vi "UploadExperiments.vi"(8 "error in (no error)":errorcluster, 11 "DB in":refnum<class "DB.lvclass">) -> (0 "error out":errorcluster, 3 "DB out":refnum<class "DB.lvclass">)   [LabVIEW 2015, in "DB.lvclass"]
uses:
  DB.lvclass
  DB.lvclass/DB.ctl
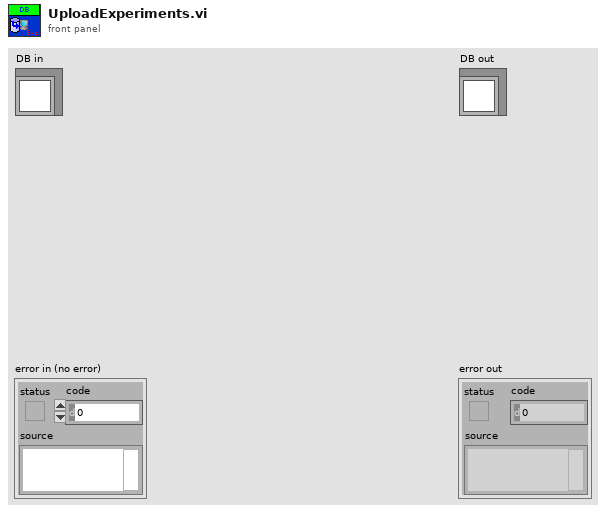
[diagram p1: front panel]
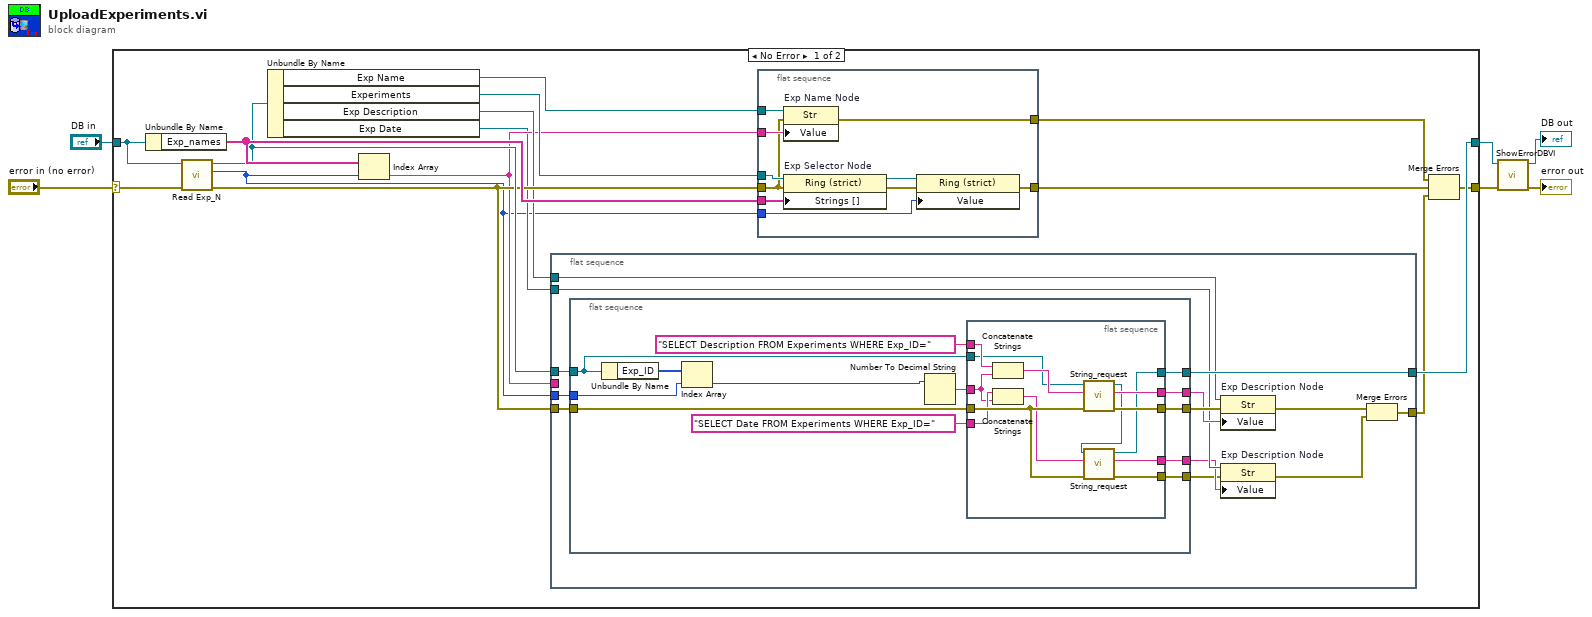
[diagram p0: block diagram]
diagram:
  n1 = case shown="No Error" "error in (no error)" {
    selector: "error in (no error)" -> [w21 w73]
    tunnel: [w14 w73] -> w6
    tunnel: [w15 w72] -> w5
    tunnel: "DB in" -> [w22 w72]
    frame No Error {
      n2 = Unbundle By Name(w22) -> ("Exp_names"=w19:string[])
      n3 = call "Read Exp_N.vi"("error in (no error)"=w21, "DB in"=w22) -> ("error out"=w13:errorcluster, "Exp_N"=w7:i16, "DB out"=w16:refnum<class "DB.lvclass">)  [unwired: 7 in]
      n4 = Unbundle By Name(w16) -> ("Exp Name"=w20:refnum<vi>, "Experiments"=w18:refnum<vi>, "Exp Description"=w12:refnum<vi>, "Exp Date"=w8:refnum<vi>)
      n5 = Index Array(array=w19, index=w7) -> (element=w9:string)
      n6 = flat-sequence {
        tunnel: w16 -> [w35]
        tunnel: [w45] -> w15
        tunnel: w13 -> [w37]
        tunnel: w12 -> [w43]
        tunnel: [w39] -> w10
        tunnel: w9 -> [_]
        tunnel: w8 -> [w41]
        tunnel: w7 -> [w34]
        frame #0 {
          n7 = flat-sequence {
            tunnel: [w58] -> w45
            tunnel: [w56] -> w44
            tunnel: [w55] -> w42
            tunnel: w37 -> [w54]
            tunnel: [w52] -> w36
            tunnel: w35 -> [w51]
            tunnel: w34 -> [w49]
            tunnel: [w46] -> w33
            frame #0 {
              n8 = Unbundle By Name(w51) -> ("Exp_ID"=w50:i16[])
              n9 = Index Array(array=w50, index=w49) -> (element=w48:i16)
              n10 = Number To Decimal String(number=w48) -> (decimal integer string=w47:string)  [unwired: 1 in]
              n11 = flat-sequence {
                tunnel: [w59] -> w58
                tunnel: "SELECT Description FROM Experiments WHERE Exp_ID=" ("SQL request") -> [w71]
                tunnel: [w69] -> w56
                tunnel: [w68] -> w55
                tunnel: w54 -> [w67]
                tunnel: "SELECT Date FROM Experiments WHERE Exp_ID=" ("SQL request") -> [w66]
                tunnel: [w64] -> w52
                tunnel: w51 -> [w63]
                tunnel: w47 -> [w62]
                tunnel: [w61] -> w46
                frame #0 {
                  n12 = Concatenate Strings(w71, w62) -> (w70:string)
                  n13 = Concatenate Strings(w66, w62) -> (w65:string)
                  n14 = call-dynamic "String_request.vi"("error in (no error)"=w67, "SQL request"=w70, "DB in"=w63) -> ("error out"=w69:errorcluster, "Result"=w68:string, "DB out"=w60:refnum<class "DB.lvclass">)  [unwired: 6 in]
                  n15 = call-dynamic "String_request.vi"("error in (no error)"=w67, "SQL request"=w65, "DB in"=w60) -> ("error out"=w61:errorcluster, "Result"=w64:string, "DB out"=w59:refnum<class "DB.lvclass">)  [unwired: 6 in]
                }
              }
            }
          }
          n16 = property on="Exp Description Node" class="Str"(reference=w43, error in=w44, "Value"=w42) -> (error out=w40:errorcluster)  [unwired: 1 out]
          n17 = property on="Exp Description Node" class="Str"(reference=w41, error in=w33, "Value"=w36) -> (error out=w38:errorcluster)  [unwired: 1 out]
          n18 = Merge Errors(w40, w38) -> (w39:errorcluster)
        }
      }
      n19 = flat-sequence {
        tunnel: w20 -> [w31]
        tunnel: w19 -> [w30]
        tunnel: w9 -> [w29]
        tunnel: w18 -> [w28]
        tunnel: [w27] -> w17
        tunnel: w7 -> [w25]
        tunnel: w13 -> [w24]
        tunnel: [w23] -> w11
        frame #0 {
          n20 = property on="Exp Name Node" class="Str"(reference=w31, error in=w24, "Value"=w29) -> (error out=w23:errorcluster)  [unwired: 1 out]
          n21 = property on="Exp Selector Node" class="Ring (strict)"(reference=w28, error in=w24, "Strings []"=w30) -> (reference out=w32:refnum<vi>, error out=w26:errorcluster)
          n22 = property class="Ring (strict)"(reference=w32, error in=w26, "Value"=w25) -> (error out=w27:errorcluster)  [unwired: 1 out]
        }
      }
      n23 = Merge Errors(w11, w17, w10) -> (w14:errorcluster)
    }
    frame Error {
    }
  }
  n24 = call "ShowErrorDBVI.vi"("error in (no error)"=w6, "DB in"=w5) -> ("error out"=→"error out":errorcluster, "DB out"=→"DB out":refnum<class "DB.lvclass">)  [unwired: 8 in]
